vi "Default Comparison Routine.vi"(10 "Person B":T1={"ID"=0, "Family Name"="Doe", "Given Name"="John", "Birth Date"=timestamp(3533142714.9178333 s since 1904-01-01)} {"Birth Date" format="%<%Y/%b/%d>T"}, 11 "Person A":T1={"ID"=0, "Family Name"="Smith", "Given Name"="John", "Birth Date"=timestamp(3533056306.0488334 s since 1904-01-01)} {"Birth Date" format="%<%Y/%b/%d>T"}) -> (3 "Swap?":bool)   [LabVIEW 2023]
doc: "This VI says that the two values should swap if Person A has a later birthday. If they have the same birthday, then they should swap if Person A has an alphabetically later name than Person B, checking last name first and then first name."
uses:
  Person Information.ctl
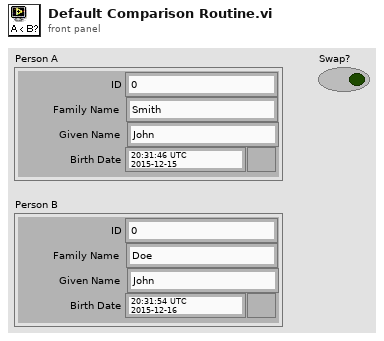
[diagram p1: front panel]
types:
  T1 = typedef "Person Information.ctl" = cluster{"ID":u32, "Family Name":string, "Given Name":string, "Birth Date":timestamp}
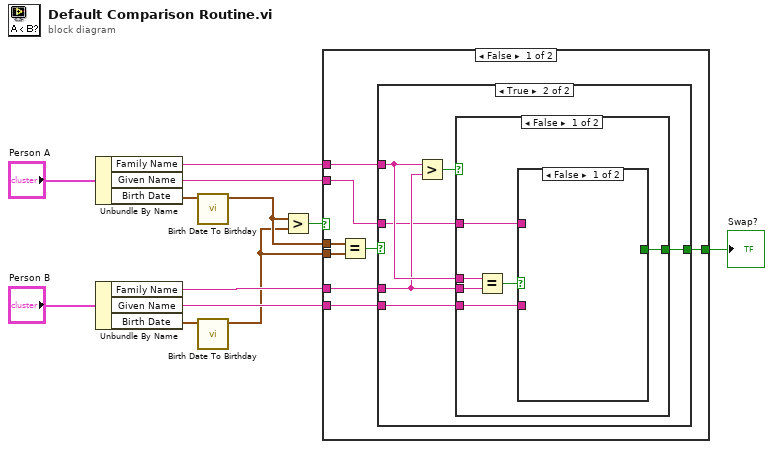
[diagram p0: block diagram]
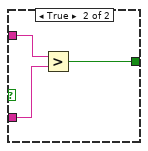
[diagram p3: hidden frame]
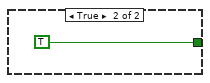
[diagram p4: hidden frame]
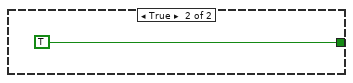
[diagram p5: hidden frame]
diagram:
  n1 = Unbundle By Name("Person A") -> ("Family Name"=w8:string, "Given Name"=w6:string, "Birth Date"=w4:timestamp)
  n2 = Unbundle By Name("Person B") -> ("Family Name"=w7:string, "Given Name"=w5:string, "Birth Date"=w2:timestamp)
  n3 = call "Birth Date To Birthday.vi"("Birth Date"=w4) -> ("Birthday"=w3:timestamp)  [unwired: 10 in]
  n4 = call "Birth Date To Birthday.vi"("Birth Date"=w2) -> ("Birthday"=w1:timestamp)  [unwired: 10 in]
  n5 = Greater?(x=w3, y=w1) -> (0:w9:bool)
  n6 = case shown="False" w9 {
    tunnel: [w15 TRUE] -> w10
    tunnel: w3 -> [w19 _]
    tunnel: w1 -> [w18 _]
    tunnel: w8 -> [w17 _]
    tunnel: w7 -> [w16 _]
    tunnel: w6 -> [w14 _]
    tunnel: w5 -> [w13 _]
    frame False {
      n7 = Equal?(x=w19, y=w18) -> (x = y?=w20:bool)
      n8 = case shown="True" w20 {
        tunnel: w17 -> [_ w24]
        tunnel: w16 -> [_ w23]
        tunnel: [_ w25] -> w15
        tunnel: w14 -> [_ w22]
        tunnel: w13 -> [_ w21]
        frame False {
        }
        frame True {
          n9 = Greater?(x=w24, y=w23) -> (0:w26:bool)
          n10 = case shown="False" w26 {
            tunnel: [w27 TRUE] -> w25
            tunnel: w24 -> [w32 _]
            tunnel: w23 -> [w31 _]
            tunnel: w22 -> [w29 _]
            tunnel: w21 -> [w28 _]
            frame False {
              n11 = Equal?(x=w32, y=w31) -> (x = y?=w30:bool)
              n12 = case shown="False" w30 {
                tunnel: w29 -> [_ w35]
                tunnel: w28 -> [_ w34]
                tunnel: [_ w33] -> w27
                frame False {
                }
                frame True {
                  n13 = Greater?(x=w35, y=w34) -> (0:w33:bool)
                }
              }
            }
            frame True {
            }
          }
        }
      }
    }
    frame True {
    }
  }
  "Swap?" <- w10
